vi "PWM CAP Get Data.vi"(8 "error in (no error)":errorcluster, 9 "pPWMData":cluster{"LowValue":u16, "HighValue":u16}, 10 "Channel":u8, 11 "DevHandle":i32) -> (0 "error out":errorcluster, 1 "pPWMData out":cluster{"LowValue":u16, "HighValue":u16}, 3 "function return":i32)   [LabVIEW 2010, in "usb2pwm.lvlib"]
doc: "int WINAPI PWM_CAP_GetData(int DevHandle, unsigned char Channel,PWM_CAP_DATA *pPWMData);"
uses:
  usb2pwm.lvlib
  libs/msvc_x86/USB2XXX.dll
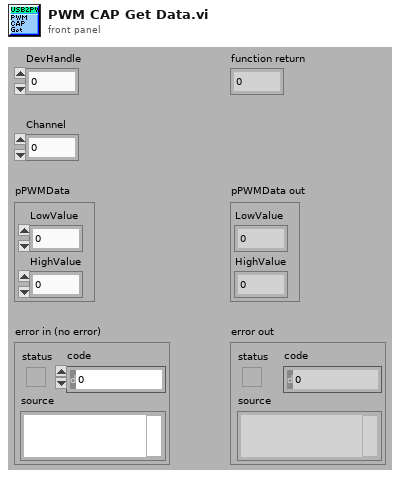
[diagram p1: front panel]
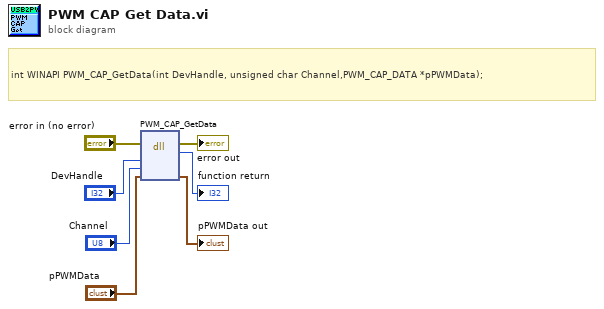
[diagram p0: block diagram]
diagram:
  # "int WINAPI PWM_CAP_GetData(int DevHandle, unsigned char Channel,PWM_CAP_DATA *pPWMData);"
  n1 = dll-call lib="E:/OtherWork/STM32/USB2XXX_Example/sdk/libs/msvc_x86/USB2XXX.*" fn="PWM_CAP_GetData"(error in="error in (no error)", "DevHandle"="DevHandle", "Channel"="Channel", "pPWMData"="pPWMData") -> (error out=→"error out":errorcluster, →"function return":i32, "pPWMData"=→"pPWMData out":cluster{"LowValue":u16, "HighValue":u16})  [unwired: 4 in, 1 out]
